vi "Read Stiffness Derived.vi"(11 "StiffnessMonitor in":refnum<class "StiffnessMonitor.lvclass">) -> (2 "Stiffness Derived":dbl[unit], 3 "StiffnessMonitor out":refnum<class "StiffnessMonitor.lvclass">)   [LabVIEW 2013, in "StiffnessMonitor.lvclass"]
uses:
  StiffnessMonitor.lvclass
  StiffnessMonitor.lvclass/StiffnessMonitor.ctl
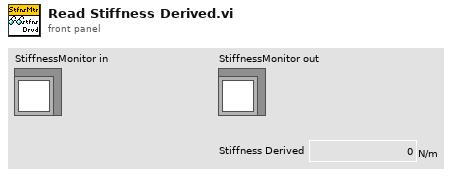
[diagram p1: front panel]
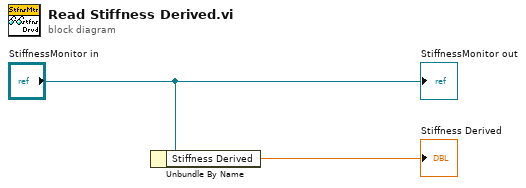
[diagram p0: block diagram]
diagram:
  n1 = Unbundle By Name("StiffnessMonitor in") -> ("Stiffness Derived"=→"Stiffness Derived":dbl[unit])
  "StiffnessMonitor out" <- "StiffnessMonitor in"
